vi "analog_read.vi"(8 "error in (no error)":errorcluster, 9 "Pin":u8=4 min=4 max=40, 11 "VISA resource name":refnum<visa-resource-name>) -> (0 "error out":errorcluster, 1 "Analog read":u16, 3 "VISA resource name out":refnum<visa-resource-name>, 6 "unsigned byte array":u8[](array[numeric]))   [LabVIEW 2025]
doc: "Este VI permite utilizar el ADC de la ESP32 para diferentes sensores \nDevuelve en valores de ADC la lectura"
panel:
  out "match substring":string
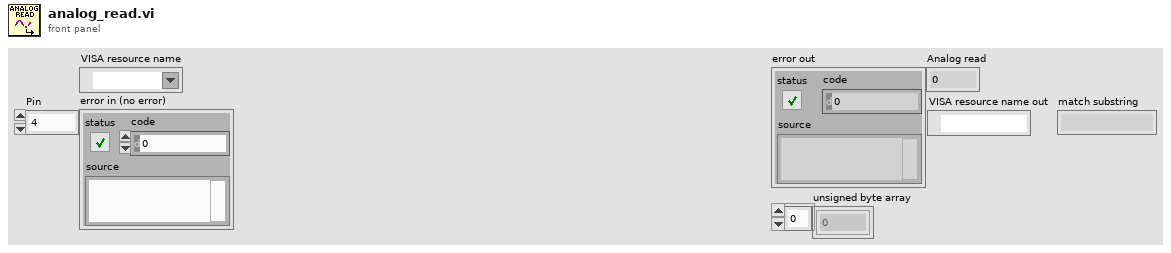
[diagram p1: front panel]
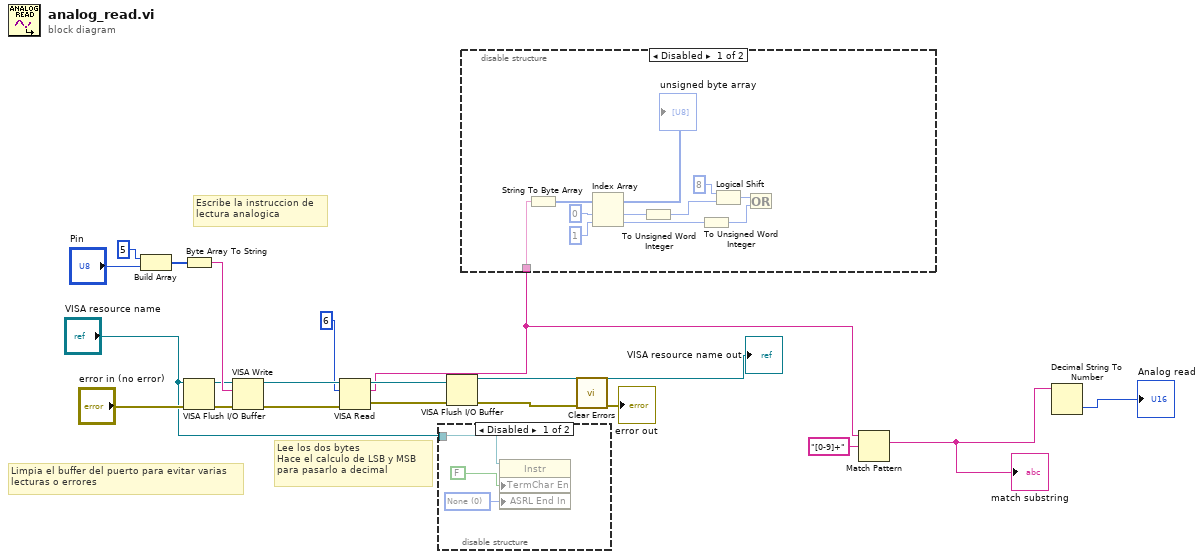
[diagram p0: block diagram]
diagram:
  # "Lee los dos bytes\nHace el calculo de LSB y MSB\npara pasarlo a decimal"
  # "Escribe la instruccion de \nlectura analogica"
  # "Limpia el buffer del puerto para evitar varias\nlecturas o errores"
  n1 = Build Array(u8 5, "Pin") -> (w18:u8[])
  n2 = Byte Array To String(unsigned byte array=w18) -> (string=w20:string)
  n3 = VISA Flush I/O Buffer(VISA resource name="VISA resource name", error in (no error)="error in (no error)") -> (VISA resource name out=w16:refnum<visa-resource-name>, error out=w15:errorcluster)  [unwired: 1 in]
  n4 = VISA Write(VISA resource name=w16, write buffer=w20, error in (no error)=w15) -> (VISA resource name out=w7:refnum<visa-resource-name>, error out=w6:errorcluster)  [unwired: 1 out]
  n5 = VISA Read(VISA resource name=w7, byte count=u32 6, error in (no error)=w6) -> (VISA resource name out=w9:refnum<visa-resource-name>, read buffer=w4:string, error out=w10:errorcluster)  [unwired: 1 out]
  n6 = disable-structure shown="Disabled" {
    disable-tunnel: "VISA resource name" -> [w23 _]
    frame Disabled {
      w22 = u16 0 items=["None", "Last Bit", "TermChar"] ("Serial Settings:End Mode for Reads")
      n7 = property class="Instr"(reference=w23, "TermChar En"=FALSE ("Message Based Settings:Termination Character Enable"), "ASRL End In"=w22) -> ()  [unwired: 1 in, 2 out]
    }
    frame Enabled {
    }
  }
  n8 = VISA Flush I/O Buffer(VISA resource name=w9, error in (no error)=w10) -> (VISA resource name out=→"VISA resource name out":refnum<visa-resource-name>, error out=w11:errorcluster)  [unwired: 1 in]
  n9 = disable-structure shown="Disabled" {
    disable-tunnel: w4 -> [w24 _]
    frame Disabled {
      n10 = String To Byte Array(string=w24) -> (unsigned byte array=w33:u8[])
      "unsigned byte array" <- w33
      n11 = Index Array(array=w33, index #1=0 ("index"), index #2=1 ("index")) -> (element #1=w27:u8, element #2=w28:u8)
      n12 = To Unsigned Word Integer(number=w27) -> (unsigned 16bit integer=w26:u16)
      n13 = To Unsigned Word Integer(number=w28) -> (unsigned 16bit integer=w25:u16)
      n14 = Logical Shift(y=8, x=w26) -> (x << y=w30:u16)
      n15 = Or(x=w30, y=w25) -> ()  [unwired: 1 out]
    }
    frame Enabled {
    }
  }
  n16 = call <vilib>:"Clear Errors.vi"("error in (no error)"=w11) -> ("error out"=→"error out":errorcluster)  [unwired: 5 in, 1 out]
  n17 = Match Pattern(string=w4, regular expression="[0-9]+") -> (match substring=w2:string)  [unwired: 1 in, 3 out]
  "match substring" <- w2
  n18 = Decimal String To Number(string=w2) -> (number=→"Analog read":i32)  [unwired: 2 in, 1 out]
